vi "Remote.TCP-IP Listener, Read Config.vi"(11 "Config Folder":path) -> (1 "Port":i32, 3 "Enabled":bool)   [LabVIEW 2024]
uses:
  <vilib>/Utility/config.llb/Read Key (Boolean).vi
  <vilib>/Utility/config.llb/Read Key (I32).vi
  <vilib>/KATE/Files/File Utils.lvlib
  <vilib>/Utility/config.llb/NI_LVConfig.lvlib
panel:
  out "Found":bool
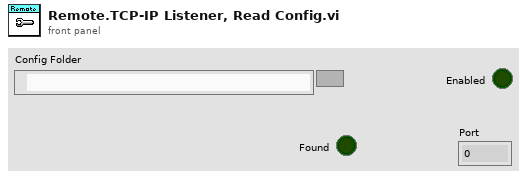
[diagram p1: front panel]
types:
  T1 = typedef "NI_LVConfig.lvlib/Config Data RefNum.ctl" = refnum<k1>
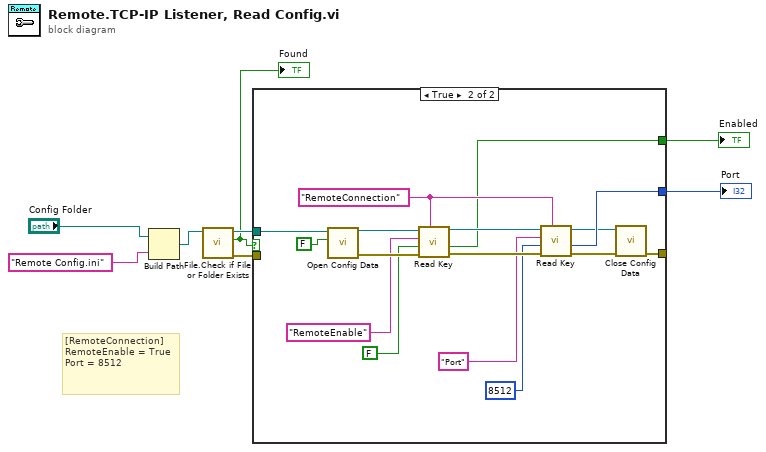
[diagram p0: block diagram]
diagram:
  # "[RemoteConnection]\nRemoteEnable = True\nPort = 8512"
  n1 = Build Path(base path="Config Folder", name or relative path="Remote Config.ini") -> (appended path=w8:path)
  n2 = call <vilib>:"File.Check if File or Folder Exists.vi"("Path"=w8) -> ("error out"=w2:errorcluster, "Exists"=w1:bool, "Dup Path"=w5:path)  [unwired: 6 in, 2 out]
  "Found" <- w1
  n3 = case shown="True" w1 {
    tunnel: w5 -> [_ w24]
    tunnel: [_ w14] -> w4
    tunnel: [_ w13] -> w3
    tunnel: [_ w9] -> _
    tunnel: w2 -> [_ _]
    frame False {
    }
    frame True {
      w19 = "RemoteConnection"
      n4 = call <vilib>:"Open Config Data.vi"("create file if necessary (T)"=FALSE, "configuration file path"=w24) -> ("error out"=w20:errorcluster, "refnum"=w22:T1)  [unwired: 7 in, 1 out]
      n5 = call-poly <vilib>:"Read Key.vi"("section"=w19, "error in (no error)"=w20, "default value"=FALSE, "key"="RemoteEnable", "refnum"=w22) -> ("error out"=w21:errorcluster, "value"=w14:bool, "refnum out"=w23:T1)  [unwired: 3 in, 1 out]
      n6 = call-poly <vilib>:"Read Key.vi"("section"=w19, "error in (no error)"=w21, "default value"=8512, "key"="Port", "refnum"=w23) -> ("error out"=w10:errorcluster, "value"=w13:i32, "refnum out"=w11:T1)  [unwired: 3 in, 1 out]
      n7 = call <vilib>:"Close Config Data.vi"("error in (no error)"=w10, "refnum"=w11) -> ("error out"=w9:errorcluster)  [unwired: 8 in, 1 out]
    }
  }
  "Enabled" <- w4
  "Port" <- w3
